vi "setTransforms.vi"(6 "transform":T1, 8 "error in (no error)":errorcluster, 11 "SceneObject in":refnum<vi>) -> (0 "error out":errorcluster, 3 "SceneObject out":refnum<vi>)   [LabVIEW 2022 SP3]
uses:
  <vilib>/picture/3D Picture Control/NI_3D Picture Control.lvlib
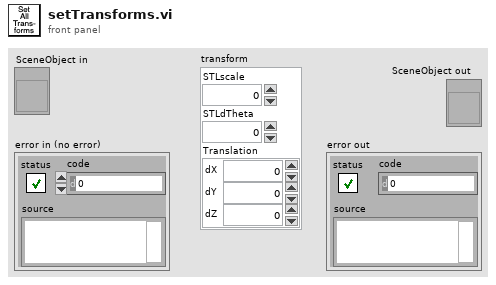
[diagram p1: front panel]
types:
  T1 = cluster{"STLscale":dbl, "STLdTheta":dbl, "Translation":cluster{"dX":sgl, "dY":sgl, "dZ":sgl}}
  T2 = cluster{"STLscale":dbl, "STLscale":dbl, "STLscale":dbl}
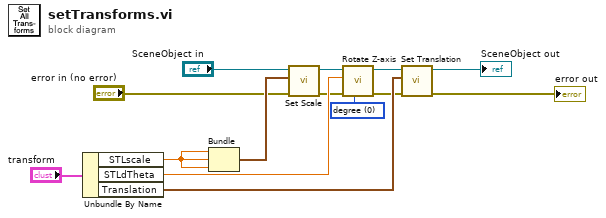
[diagram p0: block diagram]
diagram:
  w9 = u16 0 items=["degree", "radians"] ("angle unit")
  n1 = Unbundle By Name("transform") -> ("STLscale"=w6:dbl, "STLdTheta"=w11:dbl, "Translation"=w12:cluster{"dX":sgl, "dY":sgl, "dZ":sgl})
  n2 = Bundle("STLscale"=w6, "STLscale"=w6, "STLscale"=w6) -> (w5:T2)  [unwired: 1 in]
  n3 = call <vilib>:"Set Scale.vi"("error in (no error)"="error in (no error)", "Scale"=w5, "Scene Object"="SceneObject in") -> ("error out"=w3:errorcluster, "Scaled Object"=w7:refnum<vi>)  [unwired: 7 in]
  n4 = call <vilib>:"Rotate Z-axis.vi"("angle unit"=w9, "error in (no error)"=w3, "angle"=w11, "Scene Object In"=w7) -> ("error out"=w2:errorcluster, "Scene Object Out"=w8:refnum<vi>)  [unwired: 6 in]
  n5 = call <vilib>:"Set Translation.vi"("error in (no error)"=w2, "Translation"=w12, "Scene Object"=w8) -> ("error out"=→"error out":errorcluster, "Translated Object"=→"SceneObject out":refnum<vi>)  [unwired: 7 in]
